vi "Get Direction.vi"(8 "error in (no error)":errorcluster, 11 "Halfwave Sinusoidal Fit in":refnum<class "Halfwave Sinusoidal Fit.lvclass">) -> (0 "error out":errorcluster, 2 "Direction":bool, 3 "Halfwave Sinusoidal Fit out":refnum<class "Halfwave Sinusoidal Fit.lvclass">)   [LabVIEW 2013, in "Halfwave Sinusoidal Fit.lvclass"]
uses:
  Halfwave Sinusoidal Fit.lvclass
  Halfwave Sinusoidal Fit.lvclass/Halfwave Sinusoidal Fit.ctl
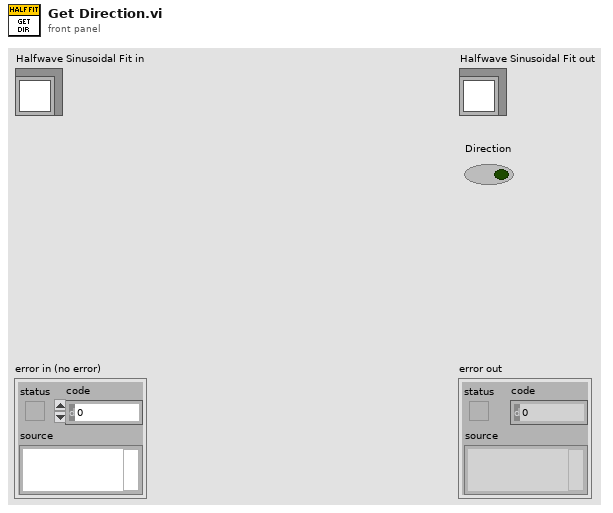
[diagram p1: front panel]
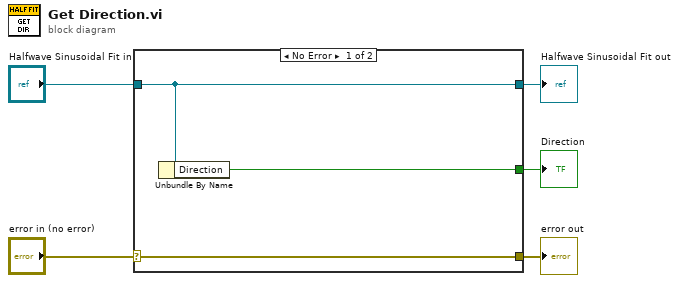
[diagram p0: block diagram]
diagram:
  n1 = case shown="No Error" "error in (no error)" {
    selector: "error in (no error)" -> [w8 w9]
    tunnel: [w8 w9] -> w4
    tunnel: [w7 w10] -> w2
    tunnel: "Halfwave Sinusoidal Fit in" -> [w7 w10]
    tunnel: [w6 _] -> w1
    frame No Error {
      n2 = Unbundle By Name(w7) -> ("Direction"=w6:bool)
    }
    frame Error {
    }
  }
  "error out" <- w4
  "Halfwave Sinusoidal Fit out" <- w2
  "Direction" <- w1
